vi "未命名 11.vi"(2 "字符串":string, 3 "初始扫描位置":u32, 4 "长度（剩余）":i32, 5 "偏移量(0)":i32) -> (0 "子字符串":string, 1 "输出 1":dbl)   [LabVIEW 2017]
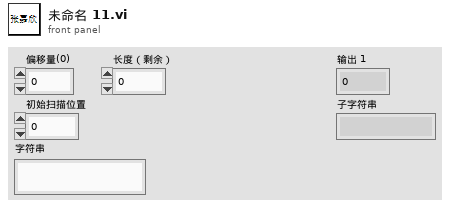
[diagram p1: front panel]
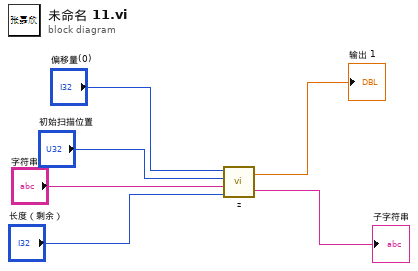
[diagram p0: block diagram]
diagram:
  n1 = call "z.vi"("长度（剩余）"="长度（剩余）", "字符串"="字符串", "初始扫描位置"="初始扫描位置", "偏移量(0)"="偏移量(0)") -> ("子字符串"=→"子字符串":string, "输出 1"=→"输出 1":dbl)
